vi "Get nx-5000 Mode.vi"(11 "IP Address":string) -> (3 "nx-5000 Mode:":string)   [LabVIEW 2019]
uses:
  <vilib>/Utility/config.llb/Read Key (String).vi
  <vilib>/FTP/NI_FTP.lvlib
  <vilib>/Utility/config.llb/NI_LVConfig.lvlib
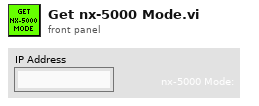
[diagram p1: front panel]
types:
  T1 = typedef "NI_LVConfig.lvlib/Config Data RefNum.ctl" = refnum<k1>
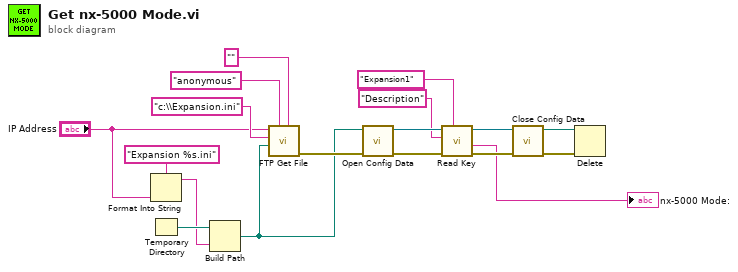
[diagram p0: block diagram]
diagram:
  n1 = Format Into String(format string="Expansion %s.ini", "IP Address") -> (resulting string=w14:string)  [unwired: 2 in, 1 out]
  n2 = Temporary Directory() -> (w17:path)
  n3 = Build Path(base path=w17, name or relative path=w14) -> (appended path=w10:path)
  n4 = call <vilib>:"FTP Get File.vi"("password"="", "user"="anonymous", "local path"=w10, "remote path"="c:\\Expansion.ini", "host"="IP Address") -> ("error out"=w11:errorcluster)  [unwired: 5 in, 1 out]
  n5 = call <vilib>:"Open Config Data.vi"("error in (no error)"=w11, "configuration file path"=w10) -> ("error out"=w8:errorcluster, "refnum"=w9:T1)  [unwired: 7 in, 1 out]
  n6 = call-poly <vilib>:"Read Key.vi"("section"="Expansion1", "error in (no error)"=w8, "key"="Description", "refnum"=w9) -> ("error out"=w4:errorcluster, "value"=→"nx-5000 Mode:":string, "refnum out"=w5:T1)  [unwired: 4 in, 1 out]
  n7 = call <vilib>:"Close Config Data.vi"("error in (no error)"=w4, "refnum"=w5) -> ("error out"=w3:errorcluster, "file path"=w2:path)  [unwired: 8 in]
  n8 = Delete(path (use dialog)=w2, error in=w3) -> ()  [unwired: 3 in, 3 out]
